vi "VI Tree.vi"   [LabVIEW 2013, in "JKI State Machine.lvlib"]
uses:
  JKI State Machine.lvlib
panel:
  # "VI TREE"
  # "For instructions on how to use the JKI State Machine, examples and video tutorials, visit:\nhttp://jkisoft.com/state-machine/\n\nJKI State Machine™\nhttp://jkisoft.com/state-machine/\nCopyright (C) 2005-2008, JKI <info@jkisoft.com>\nALL RIGHTS RESERVED"
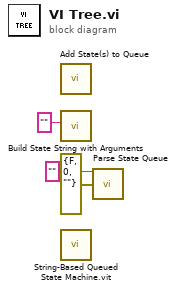
[diagram p0: block diagram]
diagram:
  n1 = call "Add State(s) to Queue.vi"() -> ()  [unwired: 15 in, 1 out]
  n2 = call "Build State String with Arguments.vi"("State"="") -> ()  [unwired: 5 in, 1 out]
  n3 = call "String-Based Queued State Machine.vit"() -> ()  [unwired: 1 in]
  n4 = call "Parse State Queue.vi"("State Queue"="", "Error In (no error)"=errorcluster {"status"=FALSE, "code"=0, "source"=""}) -> ()  [unwired: 11 in, 3 out]
